vi "Trial_Flag.vi"() -> ()   [LabVIEW 2020]
panel:
  out "Trial Flag":bool
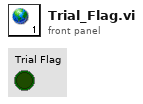
[diagram p1: front panel]
diagram:
